vi "GyroActions.vi"(10 "Update?":bool, 11 "Zero":bool) -> (0 "Fused Heading":dbl, 3 "YRPHfH":T1)   [LabVIEW 2017]
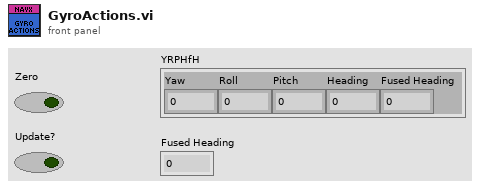
[diagram p1: front panel]
types:
  T1 = cluster{"Yaw":dbl, "Roll":dbl, "Pitch":dbl, "Heading":dbl, "Fused Heading":dbl}
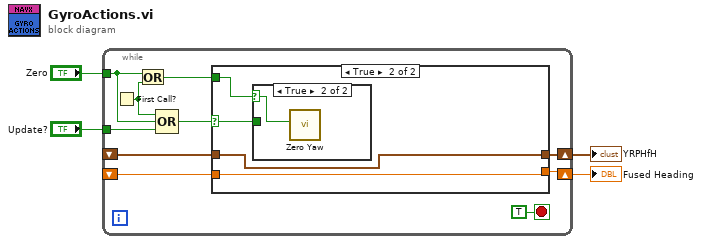
[diagram p0: block diagram]
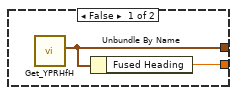
[diagram p2: hidden frame]
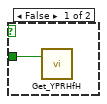
[diagram p3: hidden frame]
diagram:
  n1 = while {
    tunnel: "Update?" -> [w8]
    shift-right: [w9] -> w1
    shift-left: _ -> [w13]
    tunnel: "Zero" -> [w5]
    shift-right: [w10] -> w2
    shift-left: _ -> [w11]
    stop <- TRUE stop-if-true
    n2 = First Call?() -> (First Call?: T/F=w6:bool)
    n3 = Or(x=w5, y=w6) -> (x .or. y?=w12:bool)
    n4 = Compound Arithmetic op=OR(w6, w5, w8) -> (w7:bool)
    n5 = case shown="True" w7 {
      selector: w7 -> [_ w19]
      tunnel: w13 -> [_ w17]
      tunnel: w12 -> [_ w20]
      tunnel: w11 -> [_ w18]
      tunnel: [w16 w18] -> w10
      tunnel: [w15 w17] -> w9
      frame False {
        n6 = call <vilib>:"Get_YPRHfH.vi"() -> ("YRPHfH"=w16:T1)  [unwired: 11 in]
        n7 = Unbundle By Name(w16) -> ("Fused Heading"=w15:dbl)
      }
      frame True {
        n8 = case shown="True" w20 {
          selector: w20 -> [_ w22]
          tunnel: w19 -> [w21 _]
          frame False {
            n9 = call <vilib>:"Get_YPRHfH.vi"("Update"=w21) -> ()  [unwired: 10 in, 1 out]
          }
          frame True {
            n10 = call <vilib>:"Zero Yaw.vi"("Zero"=w22) -> ()  [unwired: 11 in]
          }
        }
      }
    }
  }
  "Fused Heading" <- w1
  "YRPHfH" <- w2
